vi "ATM Message.vi"(8 "error in":errorcluster, 10 "Index":i32) -> (0 "error IO":errorcluster, 2 "Message":string)   [LabVIEW 2013]
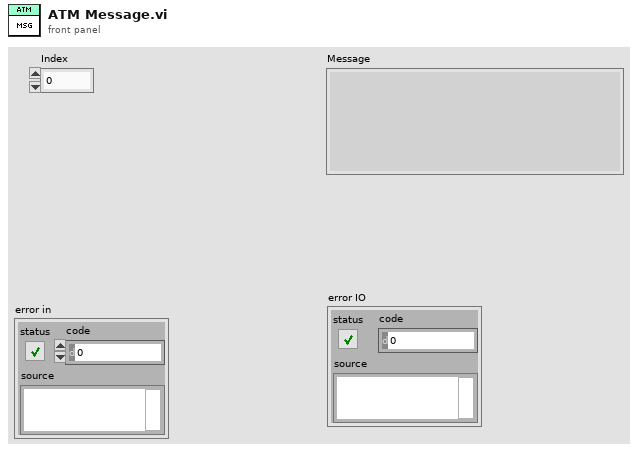
[diagram p1: front panel]
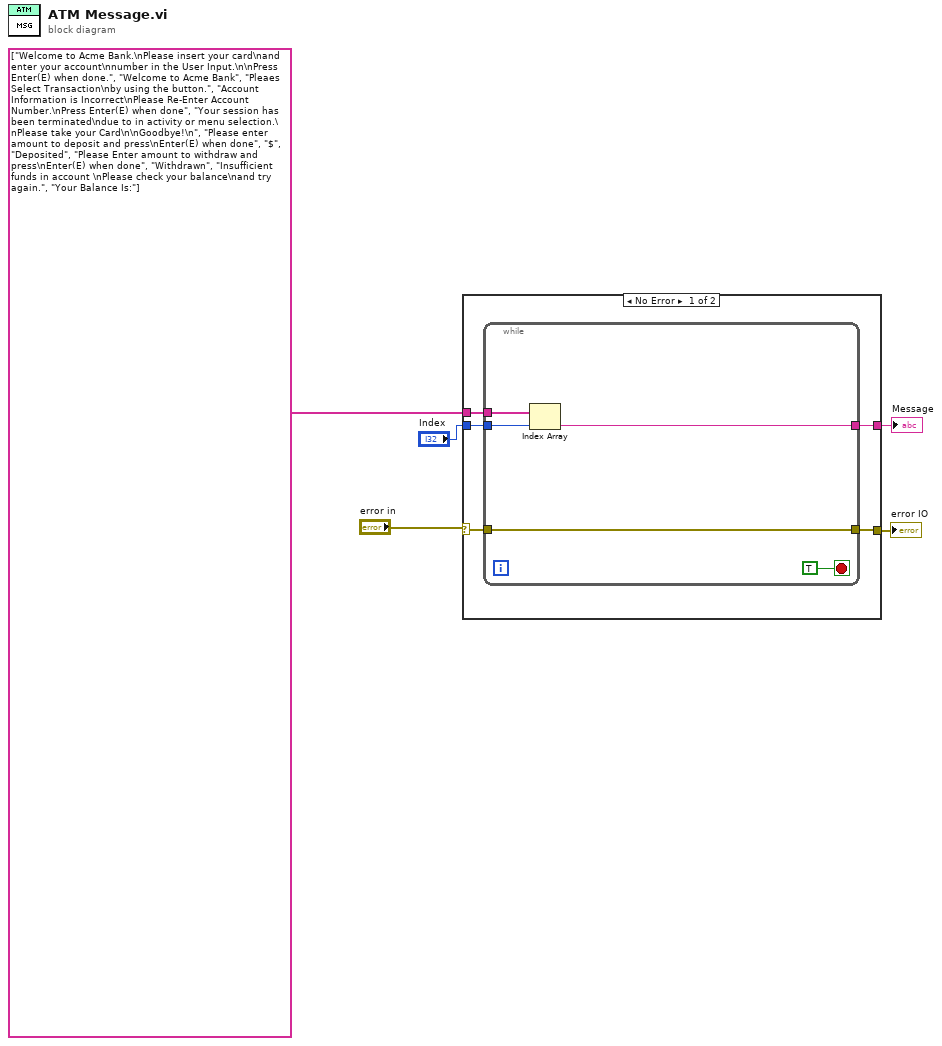
[diagram p0: block diagram]
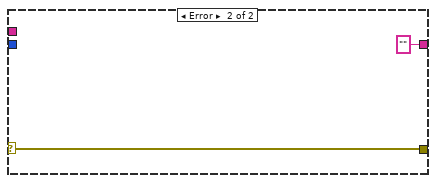
[diagram p2: hidden frame]
diagram:
  n1 = case shown="No Error" "error in" {
    selector: "error in" -> [w6 w17]
    tunnel: "Index" -> [w10 _]
    tunnel: string[] ["Welcome to Acme Bank.\nPlease insert your card\nand enter your account\nnumber in the User Input.\n\nPress Enter(E) when done.", "Welcome to Acme Bank", "Pleaes Select Transaction\nby using the button.", "Account Information is Incorrect\nPlease Re-Enter Account Number.\nPress Enter(E) when done", "Your session has been terminated\ndue to in activity or menu selection.\nPlease take your Card\n\nGoodbye!\n", "Please enter amount to deposit and press\nEnter(E) when done", "$", "Deposited", "Please Enter amount to withdraw and press\nEnter(E) when done", "Withdrawn", "Insufficient funds in account \nPlease check your balance\nand try again.", "Your Balance Is:"] -> [w9 _]
    tunnel: [w8 ""] -> w3
    tunnel: [w7 w17] -> w1
    frame No Error {
      n2 = while {
        tunnel: w10 -> [w14]
        tunnel: [w13] -> w8
        tunnel: w9 -> [w12]
        tunnel: [w11] -> w7
        tunnel: w6 -> [w11]
        stop <- TRUE stop-if-true
        n3 = Index Array(array=w12, index=w14) -> (element=w13:string)
      }
    }
    frame Error {
    }
  }
  "Message" <- w3
  "error IO" <- w1
